vi "S7_Msg_Parameters.vi"(6 "Length (bytes)":u16=1, 8 "Data Block #":u16=1, 9 "Start Address (bytes)":u32=131, 10 "Address Areas":u8(ring)=128 format="%02x" items=["I/O (P)"=128, "Input (I)"=129, "Output (Q)"=130, "Bit Memory (M)"=131, "Data (DB)"=132, "Instance Data (DI)"=133, "Local Data (L)"=134, "Predecessor Local Data (VL)"=135], 11 "Read / Write":u8(ring)=4 items=["Read"=4, "Write"=5]) -> (3 "Message Parameters":u8[](array[numeric]))   [LabVIEW 2018, in "S7 TCP.lvlib"]
uses:
  S7 TCP.lvlib
panel:
  in  "?":u16=1
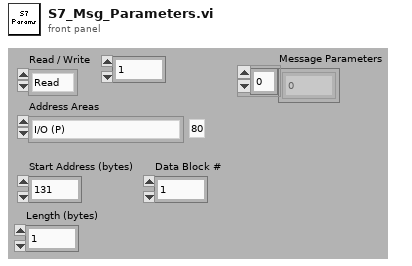
[diagram p1: front panel]
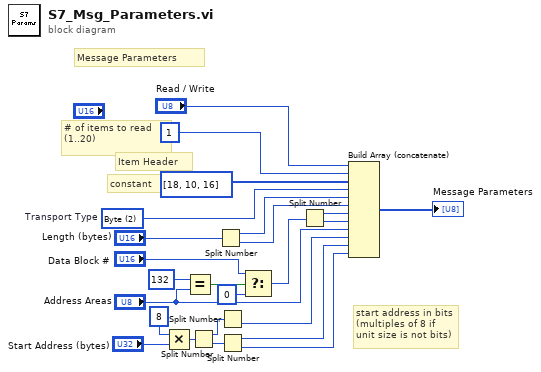
[diagram p0: block diagram]
diagram:
  w7 = u8 2 items=["Bit"=1, "Byte"=2, "Word"=4]  # Transport Type
  # "# of items to read\n(1..20)"
  # "start address in bits\n(multiples of 8 if unit size is not bits)"
  # "constant"
  # "Item Header"
  # "Message Parameters"
  n1 = Multiply(x=u32 8 ("y"), y="Start Address (bytes)") -> (x*y=w5:u32)
  n2 = Equal?(x=u8 132, y="Address Areas") -> (x = y?=w14:bool)
  n3 = Split Number(x=w5) -> (hi(x)=w22:u16, lo(x)=w21:u16)
  n4 = Split Number(x="Length (bytes)") -> (hi(x)=w18:u8, lo(x)=w6:u8)
  n5 = Split Number(x=w22) -> (lo(x)=w17:u8)  [unwired: 1 out]
  n6 = Split Number(x=w21) -> (hi(x)=w16:u8, lo(x)=w15:u8)
  n7 = Select(t="Data Block #", s=w14, f=u16 0 ("Sequence #")) -> (s? t:f=w8:u16)
  n8 = Split Number(x=w8) -> (hi(x)=w9:u8, lo(x)=w10:u8)
  n9 = Build Array (concatenate)("Read / Write", u8 1 ("Sequence #"), u8[] [18, 10, 16] ("Msg Header"), w7, w18, w6, w9, w10, "Address Areas", w17, w16, w15) -> (→"Message Parameters":u8[])
